vi "Send_Bytes.vi"(10 "Array1":u8[](array[numeric]), 11 "VISA resource name":refnum<visa-resource-name>) -> (3 "VISA resource":refnum<visa-resource-name>)   [LabVIEW 2017]
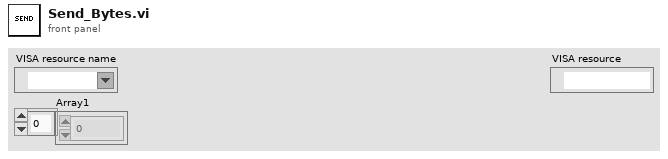
[diagram p1: front panel]
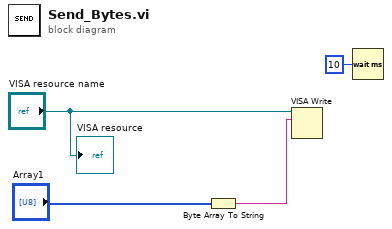
[diagram p0: block diagram]
diagram:
  n1 = Byte Array To String(unsigned byte array="Array1") -> (string=w2:string)
  n2 = VISA Write(VISA resource name="VISA resource name", write buffer=w2) -> ()  [unwired: 1 in, 3 out]
  n3 = Wait (ms)(milliseconds to wait=u32 10) -> ()  [unwired: 1 out]
  "VISA resource" <- "VISA resource name"
